vi "Test Scripting.vi"() -> ()   [LabVIEW 2011, in "Generator.lvlib"]
uses:
  Generator.lvlib
panel:
  out "x-y":u32
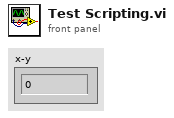
[diagram p1: front panel]
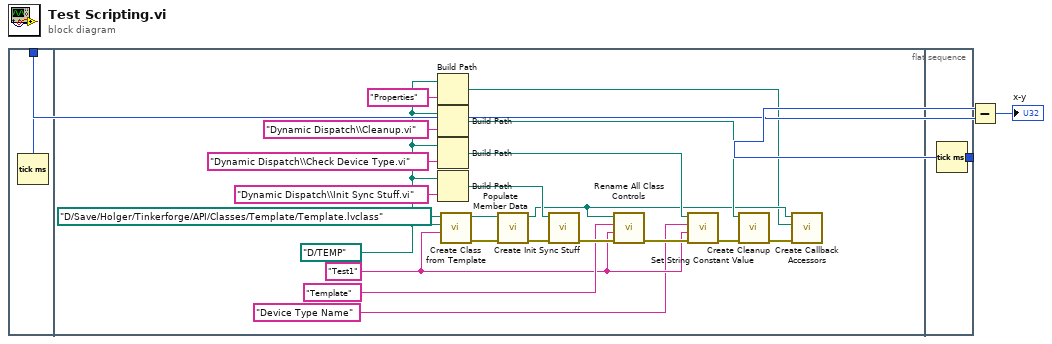
[diagram p0: block diagram]
diagram:
  n1 = flat-sequence {
    tunnel: [w4] -> w2
    tunnel: [w26] -> w3
    frame #0 {
      n2 = Tick Count (ms)() -> (millisecond timer value=w4:u32)
    }
    frame #1 {
      w14 = "Test1" ("Target Name")
      w6 = path "D:/TEMP" ("Target Path")
      n3 = Build Path(base path=w6, name or relative path="Properties") -> (appended path=w5:path)
      n4 = Build Path(base path=w6, name or relative path="Dynamic Dispatch\\Cleanup.vi") -> (appended path=w10:path)
      n5 = Build Path(base path=w6, name or relative path="Dynamic Dispatch\\Check Device Type.vi") -> (appended path=w16:path)
      n6 = Build Path(base path=w6, name or relative path="Dynamic Dispatch\\Init Sync Stuff.vi") -> (appended path=w20:path)
      n7 = call "Create Class from Template.vi"("Target Name"=w14, "Target Path"=w6, "Template Class"=path "D:/Save/Holger/Tinkerforge/API/Classes/Template/Template.lvclass") -> ("Error Out"=w24:errorcluster, "New Lib Path"=w23:path)  [unwired: 7 in]
      n8 = call "Populate Member Data.vi"("Error In"=w24, "Class Path"=w23) -> ("Error Out"=w22:errorcluster, "Class Path dup"=w8:path)  [unwired: 8 in]
      n9 = call "Create Init Sync Stuff.vi"("Error In"=w22, "File Path"=w20) -> ("Error Out"=w19:errorcluster)  [unwired: 9 in]
      n10 = call "Rename All Class Controls.vi"("Error In"=w19, "new Name"=w14, "old Name"="Template", "Class Path"=w8) -> ("Error Out"=w17:errorcluster)  [unwired: 7 in]
      n11 = call "Set String Constant Value.vi"("Error In"=w17, "Value"=w14, "Label"="Device Type Name", "VI Path"=w16) -> ("Error Out"=w12:errorcluster)  [unwired: 7 in]
      n12 = call "Create Cleanup.vi"("Error In"=w12, "File Path"=w10) -> ("Error Out"=w9:errorcluster)  [unwired: 9 in]
      n13 = call "Create Callback Accessors.vi"("Error In"=w9, "Properties Folder"=w5, "Class Path"=w8) -> ()  [unwired: 8 in, 1 out]
    }
    frame #2 {
      n14 = Tick Count (ms)() -> (millisecond timer value=w26:u32)
    }
  }
  n15 = Subtract(x=w3, y=w2) -> (x-y=→"x-y":u32)
